vi "VCS Set Ssi Abs Encoder ParameterEx.vi"(0 "axis in":cluster{"keyHandle":u32, "nodeId":u16}={"keyHandle"=0, "nodeId"=1}, 7 "SSI encoder":T1, 11 "error in (no error)":errorcluster) -> (4 "axis out":cluster{"keyHandle":u32, "nodeId":u16}={"keyHandle"=0, "nodeId"=1}, 15 "error out":errorcluster)   [LabVIEW 2017, in "maxonEPOS.lvlib"]
doc: "With function <B>VCS_SetSsiAbsEncoderParameter</B> it is possible to write all parameters for SSI absolute encoder."
uses:
  Examples/maxonEPOS.lvlib
  SSI_Tool/InstrumentsInterfaces/Motordriver/maxon EPOS/Resources/EposCmd64.dll
  SSI_Tool/InstrumentsInterfaces/Motordriver/maxon EPOS/Resources/EposCmd.dll
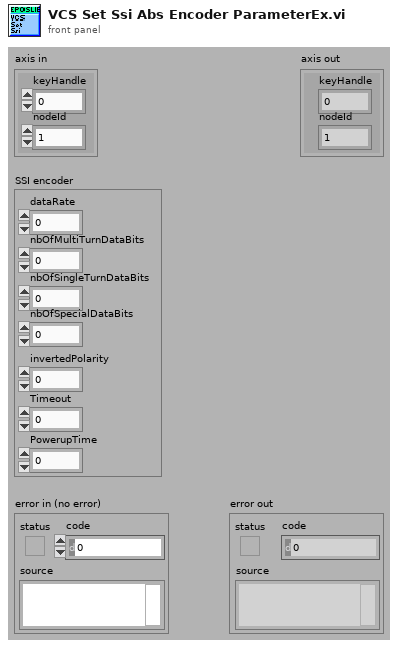
[diagram p1: front panel]
types:
  T1 = cluster{"dataRate":u16, "nbOfMultiTurnDataBits":u16, "nbOfSingleTurnDataBits":u16, "nbOfSpecialDataBits":u16, "invertedPolarity":i32, "Timeout":u16, "PowerupTime":u16}
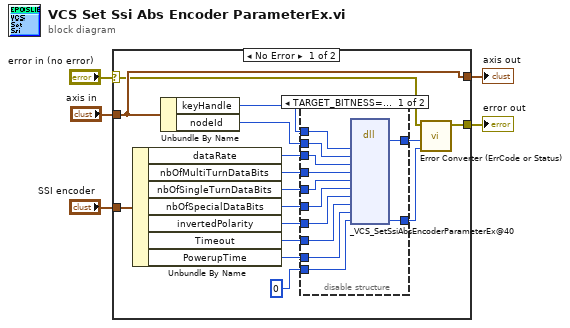
[diagram p0: block diagram]
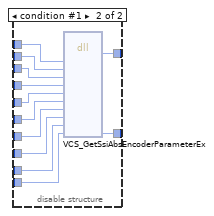
[diagram p2: hidden frame]
diagram:
  n1 = case shown="No Error" "error in (no error)" {
    selector: "error in (no error)" -> [w19 w46]
    tunnel: "axis in" -> [w21 w47]
    tunnel: [w21 w47] -> w4
    tunnel: [w20 w46] -> w3
    tunnel: "SSI encoder" -> [w15 _]
    frame No Error {
      n2 = Unbundle By Name(w15) -> ("dataRate"=w12:u16, "nbOfMultiTurnDataBits"=w11:u16, "nbOfSingleTurnDataBits"=w10:u16, "nbOfSpecialDataBits"=w9:u16, "invertedPolarity"=w8:i32, "Timeout"=w7:u16, "PowerupTime"=w6:u16)
      n3 = Unbundle By Name(w21) -> ("keyHandle"=w14:u32, "nodeId"=w13:u16)
      n4 = disable-structure shown="TARGET_BITNESS==32, Standard" {
        disable-tunnel: [w33 w35] -> w18
        disable-tunnel: [w32 w34] -> w17
        disable-tunnel: u32 0 ("pErrorCode") -> [w31 w36]
        disable-tunnel: w14 -> [w26 w45]
        disable-tunnel: w13 -> [w27 w44]
        disable-tunnel: w12 -> [w30 w43]
        disable-tunnel: w11 -> [w28 w42]
        disable-tunnel: w10 -> [w29 w41]
        disable-tunnel: w9 -> [w25 w40]
        disable-tunnel: w8 -> [w22 w39]
        disable-tunnel: w7 -> [w24 w38]
        disable-tunnel: w6 -> [w23 w37]
        frame condition #0 (active) {
          n5 = dll-call lib="C:/workspace/project/scancon/sw/SSI_Tool/InstrumentsInterfaces/Motordriver/maxon EPOS/Resources/EposCmd.*" fn="_VCS_SetSsiAbsEncoderParameterEx@40" ("EposCmd.dll:_VCS_SetSsiAbsEncoderParameter@28")("KeyHandle"=w26, "NodeId"=w27, "DataRate"=w30, "NbOfMultiTurnDataBits"=w28, "NbOfSingleTurnDataBits"=w29, "NbOfSpecialDataBits"=w25, "InvertedPolarity"=w22, "Timeout"=w24, "PowerupTime"=w23, "pErrorCode"=w31) -> ("Rückgabetyp"=w33:i32, "pErrorCode"=w32:u32)  [unwired: 12 in, 2 out]
        }
        frame condition #1 {
          n6 = dll-call lib="C:/Sources/LabVIEW/maxon EPOS/Resources/EposCmd64.dll" fn="VCS_GetSsiAbsEncoderParameterEx" ("EposCmd.dll:_VCS_SetSsiAbsEncoderParameter@28")("KeyHandle"=w45, "NodeId"=w44, "DataRate"=w43, "NbOfMultiTurnDataBits"=w42, "NbOfSingleTurnDataBits"=w41, "NbOfSpecialDataBits"=w40, "InvertedPolarity"=w39, "Timeout"=w38, "PowerupTime"=w37, "pErrorCode"=w36) -> ("Rückgabetyp"=w35:i32, "pErrorCode"=w34:u32)  [unwired: 12 in, 2 out]
        }
      }
      n7 = call "Error Converter (ErrCode or Status).vi"("error code"=w17, "return type"=w18, "error in (no error)"=w19) -> ("error out"=w20:errorcluster)  [unwired: 7 in]
    }
    frame Error {
    }
  }
  "error out" <- w3
  "axis out" <- w4
